vi "FilterLittle_Location.vi"(10 "UTM Location":T1 {"North" format="%#_10f"; "East" format="%#_8f"}, 11 "Notifier in":refnum<notifier>) -> ()   [LabVIEW 2013]
doc: "If the location of the little boat is less than zero (that test case should really be done with whatever the GPS writes when it can't find a match, perhaps -1) the latest GPS data is not written up into other areas of the boat like MidBrain. It is not passed into the BoatLocation notifier.\n\nEric Schneider, April 2014"
uses:
  Data/TypeDefs/UTM Location.ctl
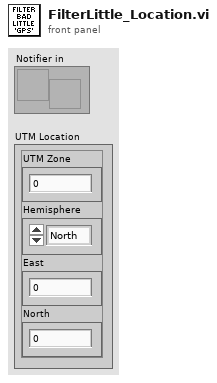
[diagram p1: front panel]
types:
  T1 = typedef "UTM Location.ctl" = cluster{"UTM Zone":dbl, "Hemisphere":enum16{"North", "South"}, "East":dbl, "North":dbl}
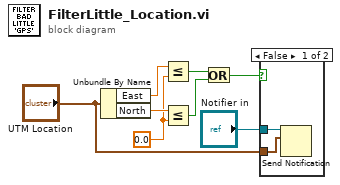
[diagram p0: block diagram]
diagram:
  w5 = 0.0 ("y")
  n1 = Unbundle By Name("UTM Location") -> ("East"=w7:dbl, "North"=w6:dbl)
  n2 = Less Or Equal?(x=w7, y=w5) -> (x <= y?=w4:bool)
  n3 = Less Or Equal?(x=w6, y=w5) -> (x <= y?=w3:bool)
  n4 = Or(x=w4, y=w3) -> (x .or. y?=w2:bool)
  n5 = case shown="False" w2 {
    tunnel: "Notifier in" -> [w10 _]
    tunnel: "UTM Location" -> [w9 _]
    frame False {
      n6 = Send Notification(notification=w9, notifier=w10) -> ()  [unwired: 1 in, 2 out]
    }
    frame True {
    }
  }
